vi "Main.vi"() -> ()   [LabVIEW 2019]
uses:
  Type defs/Elevator position.ctl
  Type defs/Car buttons.ctl
  Type defs/Main states.ctl
  Type defs/Elevator states.ctl
panel:
  in  "Select mode":bool
  in  "Floor array":cluster{"Up Button":bool, "Down Button":bool}[](array[cluster])
  in  "E4":T1
  in  "E3":T1
  in  "E2":T1
  in  "E1":T1
  in  "stop":bool
  # "20"
  # "19"
  # "18"
  # "17"
  # "16"
  # "15"
  # "14"
  # "13"
  # "12"
  # "11"
  # "10"
  # "9"
  # "8"
  # "7"
  # "6"
  # "5"
  # "4"
  # "3"
  # "2"
  # "1"
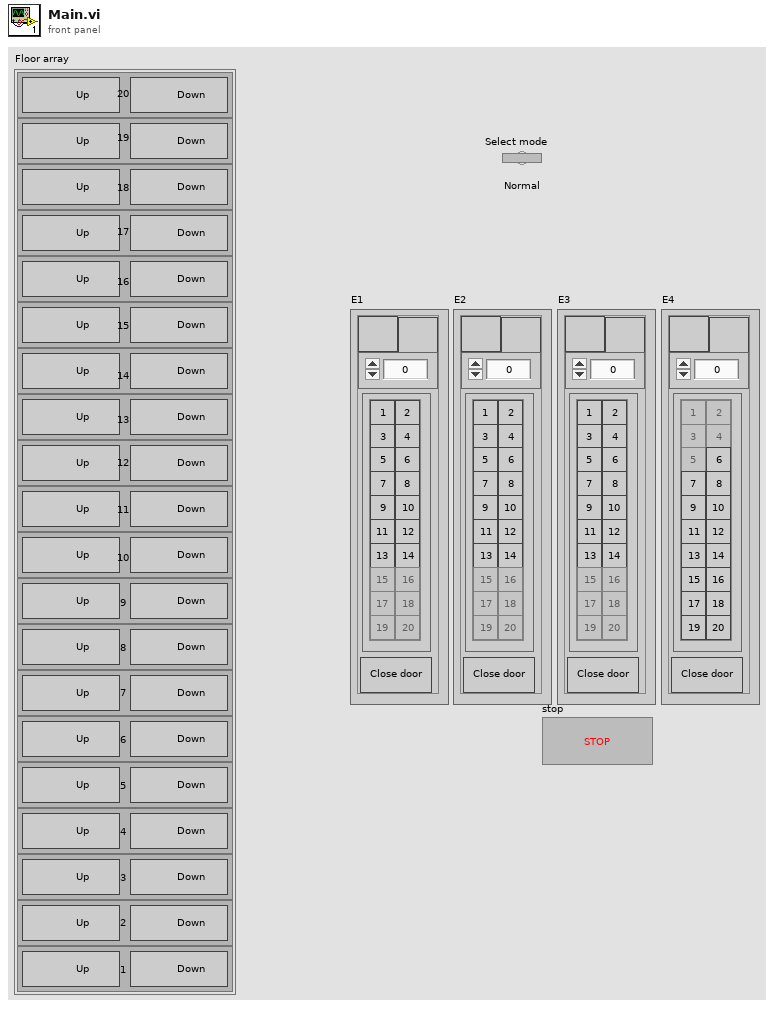
[diagram p1: front panel]
types:
  T1 = typedef "Elevator position.ctl" = cluster{"Up Button":bool, "Current floor":u16, "Down Button":bool, "Car":T2, "Close door":bool}
  T2 = typedef "Car buttons.ctl" = cluster{"Blank Button":bool, "Blank Button 2":bool, "Blank Button 3":bool, "Blank Button 4":bool, "Blank Button 5":bool, "Blank Button 6":bool, "Blank Button 7":bool, "Blank Button 8":bool, "Blank Button 9":bool, "Blank Button 10":bool, "Blank Button 11":bool, "Blank Button 12":bool, "Blank Button 13":bool, "Blank Button 14":bool, "Blank Button 15":bool, "Blank Button 16":bool, "Blank Button 17":bool, "Blank Button 18":bool, "Blank Button 19":bool, "Blank Button 20":bool}
  T3 = typedef "Main states.ctl" = enum16{"Init", "GUI", "Check next destination", "Move elevator", "Wait button press", "End"}
  T4 = typedef "Elevator states.ctl" = cluster{"Elevator":T1, "Destinations":i32[], "Idle floor":u16, "Max floor":u16, "Min floor":u16, "Next floor":u16, "Move started":timestamp, "Idle move":bool}
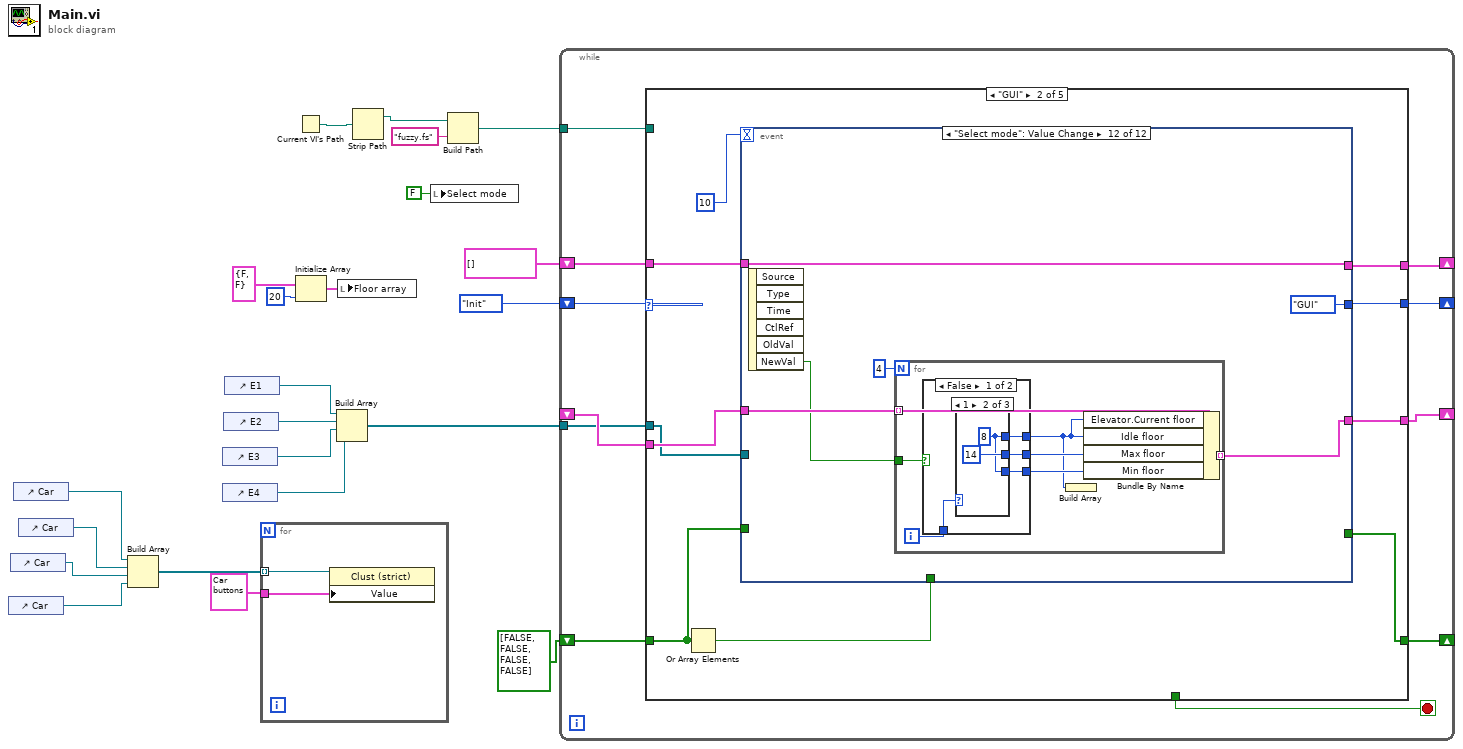
[diagram p0: block diagram]
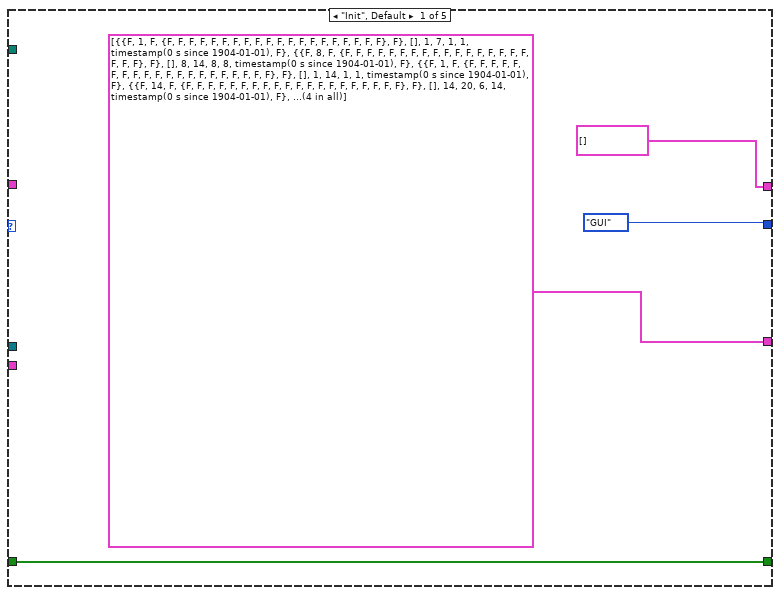
[diagram p2: hidden frame]
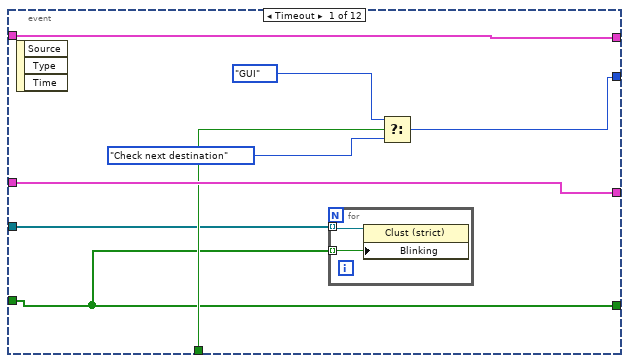
[diagram p3: hidden frame]
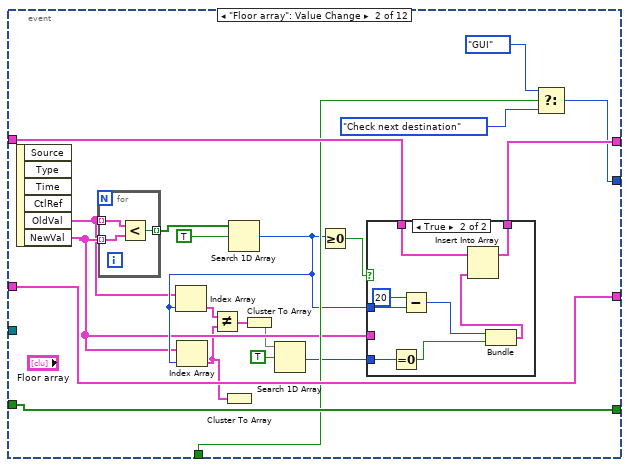
[diagram p4: hidden frame]
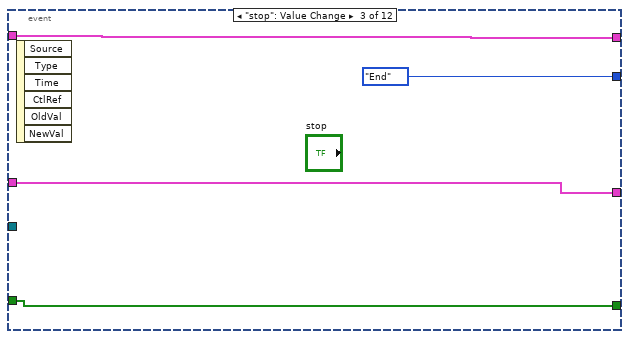
[diagram p6: hidden frame]
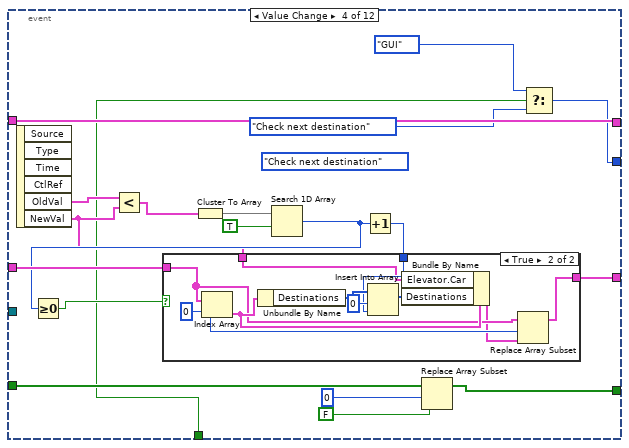
[diagram p7: hidden frame]
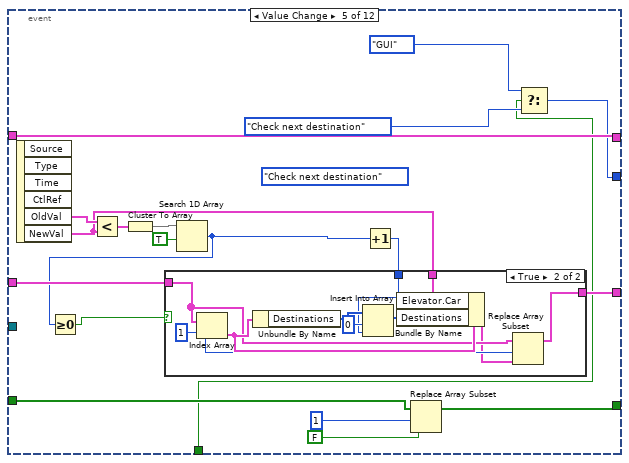
[diagram p9: hidden frame]
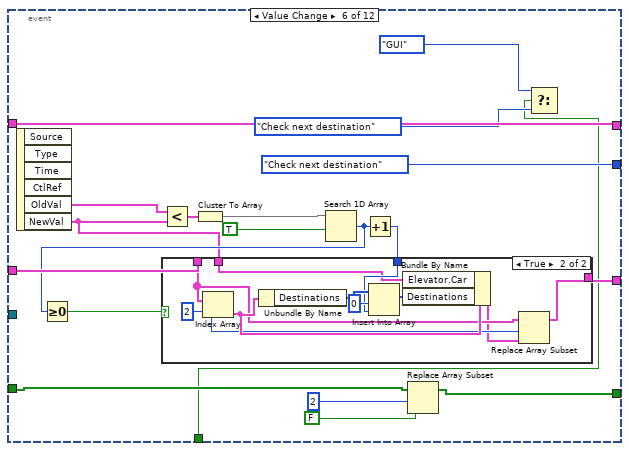
[diagram p11: hidden frame]
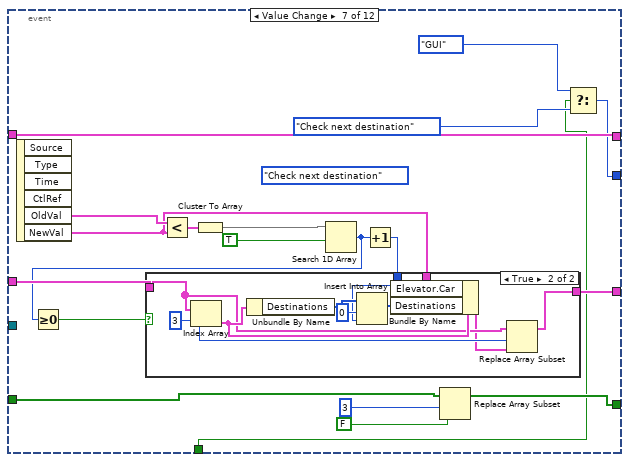
[diagram p13: hidden frame]
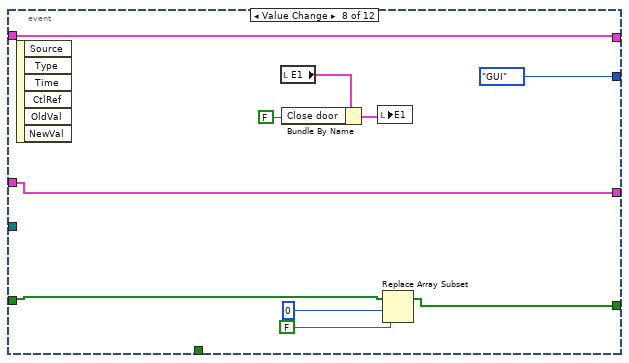
[diagram p15: hidden frame]
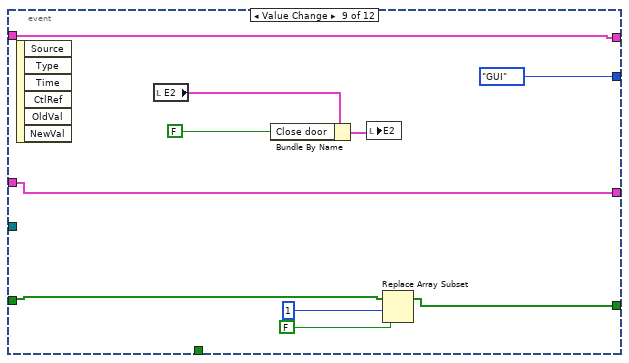
[diagram p16: hidden frame]
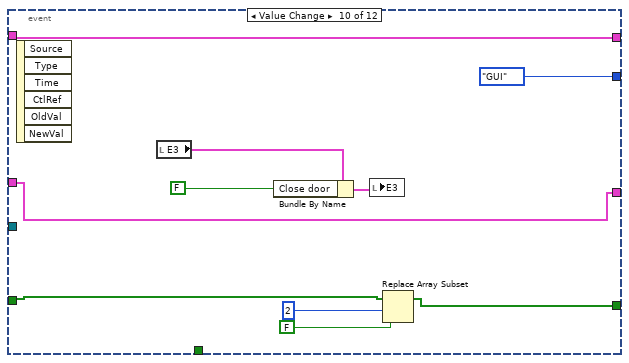
[diagram p17: hidden frame]
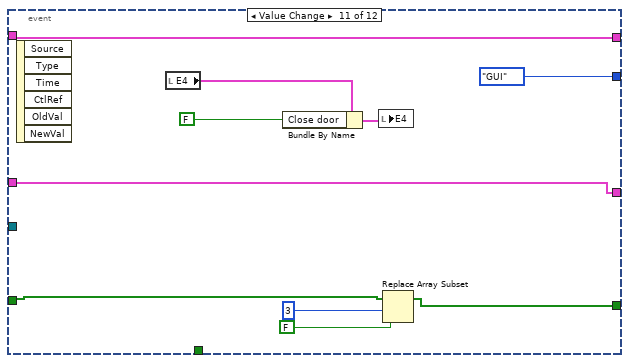
[diagram p18: hidden frame]
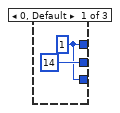
[diagram p19: hidden frame]
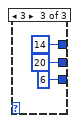
[diagram p20: hidden frame]
diagram:
  n1 = control-ref of="Car"() -> (w3:refnum<vi>)
  n2 = control-ref of="Car"() -> (w4:refnum<vi>)
  n3 = control-ref of="Car"() -> (w6:refnum<vi>)
  n4 = control-ref of="Car"() -> (w5:refnum<vi>)
  n5 = Build Array(w6, w5, w4, w3) -> (w2:refnum<vi>[])
  n6 = control-ref of="E3"() -> (w18:refnum<vi>)
  n7 = control-ref of="E4"() -> (w17:refnum<vi>)
  n8 = control-ref of="E2"() -> (w19:refnum<vi>)
  n9 = control-ref of="E1"() -> (w20:refnum<vi>)
  n10 = for {
    tunnel: T2 {"Blank Button"=FALSE, "Blank Button 2"=FALSE, "Blank Button 3"=FALSE, "Blank Button 4"=FALSE, "Blank Button 5"=FALSE, "Blank Button 6"=FALSE, "Blank Button 7"=FALSE, "Blank Button 8"=FALSE, "Blank Button 9"=FALSE, "Blank Button 10"=FALSE, "Blank Button 11"=FALSE, "Blank Button 12"=FALSE, "Blank Button 13"=FALSE, "Blank Button 14"=FALSE, "Blank Button 15"=FALSE, "Blank Button 16"=FALSE, "Blank Button 17"=FALSE, "Blank Button 18"=FALSE, "Blank Button 19"=FALSE, "Blank Button 20"=FALSE} ("Value") -> [w24]
    tunnel: w2 -> [w23] mode=indexing
    n11 = property class="Clust (strict)"(reference=w23, "Value"=w24) -> ()  [unwired: 1 in, 2 out]
  }
  n12 = Current VI's Path() -> (path=w12:path)
  n13 = Initialize Array(cluster{"Up Button":bool, "Down Button":bool} {"Up Button"=FALSE, "Down Button"=FALSE} ("Cluster"), 20 ("dimension size")) -> (w8:cluster{"Up Button":bool, "Down Button":bool}[])
  n14 = Build Array(w20, w19, w18, w17) -> (w16:refnum<vi>[])
  n15 = local write "Floor array"(w8) -> ()
  n16 = Strip Path(path=w12) -> (stripped path=w13:path)  [unwired: 1 out]
  n17 = local write "Select mode"(FALSE ("Select mode")) -> ()
  n18 = Build Path(base path=w13, name or relative path="fuzzy.fs") -> (appended path=w11:path)
  n19 = while {
    shift-right: [w34] -> _
    shift-left: cluster{"H call":dbl, "Up":bool}[] [] ("Array") -> [w33]
    shift-right: [w30] -> _
    shift-left: Main_states."Init" -> [w35]
    shift-right: [w29] -> _
    shift-left: _ -> [w32]
    tunnel: w16 -> [w28]
    shift-right: [w27] -> _
    shift-left: bool[] [FALSE, FALSE, FALSE, FALSE] ("Served car") -> [w26]
    tunnel: w11 -> [w25]
    stop <- w31 stop-if-true
    n20 = case shown="\"GUI\"" w35 {
      tunnel: [cluster{"H call":dbl, "Up":bool}[] [] ("Array") w48 w295 w327 w351] -> w34
      tunnel: w33 -> [_ w47 w296 w327 w351]
      tunnel: [Main_states."GUI" w46 Main_states."Move elevator" Main_states."GUI" Main_states."End"] -> w30
      tunnel: [T4[] [{"Elevator"={"Up Button"=FALSE, "Current floor"=1, "Down Button"=FALSE, "Car"={"Blank Button"=FALSE, "Blank Button 2"=FALSE, "Blank Button 3"=FALSE, "Blank Button 4"=FALSE, "Blank Button 5"=FALSE, "Blank Button 6"=FALSE, "Blank Button 7"=FALSE, "Blank Button 8"=FALSE, "Blank Button 9"=FALSE, "Blank Button 10"=FALSE, "Blank Button 11"=FALSE, "Blank Button 12"=FALSE, "Blank Button 13"=FALSE, "Blank Button 14"=FALSE, "Blank Button 15"=FALSE, "Blank Button 16"=FALSE, "Blank Button 17"=FALSE, "Blank Button 18"=FALSE, "Blank Button 19"=FALSE, "Blank Button 20"=FALSE}, "Close door"=FALSE}, "Destinations"=[], "Idle floor"=1, "Max floor"=7, "Min floor"=1, "Next floor"=1, "Move started"=timestamp(0 s since 1904-01-01), "Idle move"=FALSE}, {"Elevator"={"Up Button"=FALSE, "Current floor"=8, "Down Button"=FALSE, "Car"={"Blank Button"=FALSE, "Blank Button 2"=FALSE, "Blank Button 3"=FALSE, "Blank Button 4"=FALSE, "Blank Button 5"=FALSE, "Blank Button 6"=FALSE, "Blank Button 7"=FALSE, "Blank Button 8"=FALSE, "Blank Button 9"=FALSE, "Blank Button 10"=FALSE, "Blank Button 11"=FALSE, "Blank Button 12"=FALSE, "Blank Button 13"=FALSE, "Blank Button 14"=FALSE, "Blank Button 15"=FALSE, "Blank Button 16"=FALSE, "Blank Button 17"=FALSE, "Blank Button 18"=FALSE, "Blank Button 19"=FALSE, "Blank Button 20"=FALSE}, "Close door"=FALSE}, "Destinations"=[], "Idle floor"=8, "Max floor"=14, "Min floor"=8, "Next floor"=8, "Move started"=timestamp(0 s since 1904-01-01), "Idle move"=FALSE}, {"Elevator"={"Up Button"=FALSE, "Current floor"=1, "Down Button"=FALSE, "Car"={"Blank Button"=FALSE, "Blank Button 2"=FALSE, "Blank Button 3"=FALSE, "Blank Button 4"=FALSE, "Blank Button 5"=FALSE, "Blank Button 6"=FALSE, "Blank Button 7"=FALSE, "Blank Button 8"=FALSE, "Blank Button 9"=FALSE, "Blank Button 10"=FALSE, "Blank Button 11"=FALSE, "Blank Button 12"=FALSE, "Blank Button 13"=FALSE, "Blank Button 14"=FALSE, "Blank Button 15"=FALSE, "Blank Button 16"=FALSE, "Blank Button 17"=FALSE, "Blank Button 18"=FALSE, "Blank Button 19"=FALSE, "Blank Button 20"=FALSE}, "Close door"=FALSE}, "Destinations"=[], "Idle floor"=1, "Max floor"=14, "Min floor"=1, "Next floor"=1, "Move started"=timestamp(0 s since 1904-01-01), "Idle move"=FALSE}, {"Elevator"={"Up Button"=FALSE, "Current floor"=14, "Down Button"=FALSE, "Car"={"Blank Button"=FALSE, "Blank Button 2"=FALSE, "Blank Button 3"=FALSE, "Blank Button 4"=FALSE, "Blank Button 5"=FALSE, "Blank Button 6"=FALSE, "Blank Button 7"=FALSE, "Blank Button 8"=FALSE, "Blank Button 9"=FALSE, "Blank Button 10"=FALSE, "Blank Button 11"=FALSE, "Blank Button 12"=FALSE, "Blank Button 13"=FALSE, "Blank Button 14"=FALSE, "Blank Button 15"=FALSE, "Blank Button 16"=FALSE, "Blank Button 17"=FALSE, "Blank Button 18"=FALSE, "Blank Button 19"=FALSE, "Blank Button 20"=FALSE}, "Close door"=FALSE}, "Destinations"=[], "Idle floor"=14, "Max floor"=20, "Min floor"=6, "Next floor"=14, "Move started"=timestamp(0 s since 1904-01-01), "Idle move"=FALSE}] ("Elevator states array") w44 w294 w312 w350] -> w29
      tunnel: w32 -> [_ w45 w293 w325 w350]
      tunnel: [_ _ _ _ TRUE] -> w31
      tunnel: w28 -> [_ w40 _ _ _]
      tunnel: [w36 w41 w291 w309 w347] -> w27
      tunnel: w26 -> [w36 w42 w291 _ w347]
      tunnel: w25 -> [_ _ w289 _ _]
      frame "Init", Default {
      }
      frame "GUI" {
        n21 = Or Array Elements(Boolean array=w42) -> (logical OR=w43:bool)
        n22 = event shown="[11] \"Select mode\": Value Change" {
          selector: _ -> [_ _ _ _ _ _ _ _ _ _ _ _]
          dyn-events: _ -> [_ _ _ _ _ _ _ _ _ _ _ _]
          timeout: 10 -> [_ _ _ _ _ _ _ _ _ _ _ _]
          tunnel: [w57 w75 w95 w110 w140 w170 w200 w218 w228 w237 w251 w260] -> w48
          tunnel: w47 -> [w57 w76 w95 w110 w140 w170 w200 w218 w228 w237 w251 w260]
          tunnel: [w53 w70 Main_states."End" w96 w127 Main_states."Check next destination" w187 Main_states."GUI" Main_states."GUI" Main_states."GUI" Main_states."GUI" Main_states."GUI"] -> w46
          tunnel: w45 -> [w56 w79 w93 w108 w138 w167 w198 w217 w226 w238 w250 w259]
          tunnel: [w56 w79 w93 w107 w137 w166 w197 w217 w226 w238 w250 w257] -> w44
          tunnel: w43 -> [w55 w71 _ w97 w128 w157 w188 _ _ _ _ _]
          tunnel: w42 -> [w50 w74 w92 w103 w132 w161 w192 w223 w233 w243 w253 _]
          tunnel: [w50 w74 w92 w100 w131 w160 w191 w222 w232 w242 w252 _] -> w41
          tunnel: w40 -> [w51 _ _ _ _ _ _ _ _ _ _ _]
          event Timeout {
            n23 = event-data() -> ()  [unwired: 1 in, 3 out]
            n24 = for {
              tunnel: w51 -> [w59] mode=indexing
              tunnel: w50 -> [w58] mode=indexing
              n25 = property class="Clust (strict)"(reference=w59, "Blinking"=w58) -> ()  [unwired: 1 in, 2 out]
            }
            n26 = Select(t=Main_states."GUI", s=w55, f=Main_states."Check next destination") -> (s? t:f=w53:T3)
          }
          event "Floor array": Value Change {
            n27 = event-data() -> ("OldVal"=w63:cluster{"Up Button":bool, "Down Button":bool}[], "NewVal"=w68:cluster{"Up Button":bool, "Down Button":bool}[])  [unwired: 1 in, 4 out]
            n28 = for {
              tunnel: w63 -> [w91] mode=indexing
              tunnel: w68 -> [w90] mode=indexing
              tunnel: [w89] -> w78 mode=indexing
              n29 = Less?(x=w91, y=w90) -> (x < y?=w89:bool)
            }
            n30 = Search 1D Array(1D array=w78, element=TRUE) -> (index of element=w69:i32)  [unwired: 1 in]
            n31 = Index Array(array=w63, index=w69) -> (element=w67:cluster{"Up Button":bool, "Down Button":bool})
            n32 = Index Array(array=w68, index=w69) -> (element=w61:cluster{"Up Button":bool, "Down Button":bool})
            n33 = Not Equal?(x=w67, y=w61) -> (x != y?=w66:cluster{"Up Button":bool, "Down Button":bool})
            n34 = Cluster To Array(cluster=w61) -> ()  [unwired: 1 out]
            n35 = Cluster To Array(cluster=w66) -> (array=w62:bool[])
            n36 = Search 1D Array(1D array=w62, element=TRUE) -> (index of element=w60:i32)  [unwired: 1 in]
            n37 = Greater Or Equal To 0?(x=w69) -> (x >= 0?=w77:bool)
            n38 = case shown="True" w77 {
              tunnel: w69 -> [_ w88]
              tunnel: w76 -> [w80 w86]
              tunnel: [w80 w85] -> w75
              tunnel: w68 -> [_ _]
              tunnel: w60 -> [_ w82]
              frame False {
              }
              frame True {
                n39 = Equal To 0?(x=w82) -> (x = 0?=w81:bool)
                n40 = Subtract(x=20, y=w88) -> (x-y=w84:i32)
                n41 = Bundle(w84, w81) -> (w83:cluster{i32, bool})  [unwired: 1 in]
                n42 = Insert Into Array(array=w86, new element=w83) -> (w85:cluster{"H call":dbl, "Up":bool}[])  [unwired: 1 in]
              }
            }
            n43 = Select(t=Main_states."GUI", s=w71, f=Main_states."Check next destination") -> (s? t:f=w70:T3)
          }
          event "stop": Value Change {
            n44 = event-data() -> ()  [unwired: 1 in, 6 out]
          }
          event Value Change {
            (unwired) Main_states."Check next destination"
            n45 = event-data() -> ("OldVal"=w111:T2, "NewVal"=w104:T2)  [unwired: 1 in, 4 out]
            n46 = Less?(x=w111, y=w104) -> (x < y?=w114:T2)
            n47 = Cluster To Array(cluster=w114) -> (array=w113:bool[])
            n48 = Search 1D Array(1D array=w113, element=TRUE) -> (index of element=w106:i32)  [unwired: 1 in]
            n49 = Greater Or Equal To 0?(x=w106) -> (x >= 0?=w105:bool)
            n50 = Increment(x=w106) -> (x+1=w109:i32)
            n51 = case shown="True" w105 {
              tunnel: w109 -> [_ w122]
              tunnel: w108 -> [w115 w120]
              tunnel: [w115 w117] -> w107
              tunnel: w104 -> [_ w116]
              frame False {
              }
              frame True {
                w119 = 0 ("index")
                n52 = Index Array(array=w120, index=w119) -> (element=w125:T4)
                n53 = Unbundle By Name(w125) -> ("Destinations"=w124:i32[])
                n54 = Insert Into Array(array=w124, index=0, new element=w122) -> (w121:i32[])
                n55 = Bundle By Name(cluster=w125, "Elevator.Car"=w116, "Destinations"=w121) -> (w118:T4)
                n56 = Replace Array Subset(array=w120, new element=w118, index=w119) -> (w117:T4[])
              }
            }
            n57 = Replace Array Subset(array=w103, new element=FALSE ("new element/subarray"), index=0) -> (w100:bool[])
            n58 = Select(t=Main_states."GUI", s=w97, f=Main_states."Check next destination") -> (s? t:f=w96:T3)
          }
          event Value Change {
            (unwired) Main_states."Check next destination"
            n59 = event-data() -> ("OldVal"=w141:T2, "NewVal"=w126:T2)  [unwired: 1 in, 4 out]
            n60 = Less?(x=w141, y=w126) -> (x < y?=w144:T2)
            n61 = Cluster To Array(cluster=w144) -> (array=w143:bool[])
            n62 = Search 1D Array(1D array=w143, element=TRUE) -> (index of element=w136:i32)  [unwired: 1 in]
            n63 = Greater Or Equal To 0?(x=w136) -> (x >= 0?=w135:bool)
            n64 = Increment(x=w136) -> (x+1=w139:i32)
            n65 = case shown="True" w135 {
              tunnel: w139 -> [_ w152]
              tunnel: w138 -> [w145 w150]
              tunnel: [w145 w147] -> w137
              tunnel: w126 -> [_ w146]
              frame False {
              }
              frame True {
                w149 = 1 ("index")
                n66 = Index Array(array=w150, index=w149) -> (element=w155:T4)
                n67 = Unbundle By Name(w155) -> ("Destinations"=w154:i32[])
                n68 = Insert Into Array(array=w154, index=0, new element=w152) -> (w151:i32[])
                n69 = Bundle By Name(cluster=w155, "Elevator.Car"=w146, "Destinations"=w151) -> (w148:T4)
                n70 = Replace Array Subset(array=w150, new element=w148, index=w149) -> (w147:T4[])
              }
            }
            n71 = Replace Array Subset(array=w132, new element=FALSE ("new element/subarray"), index=1) -> (w131:bool[])
            n72 = Select(t=Main_states."GUI", s=w128, f=Main_states."Check next destination") -> (s? t:f=w127:T3)
          }
          event Value Change {
            n73 = event-data() -> ("OldVal"=w171:T2, "NewVal"=w156:T2)  [unwired: 1 in, 4 out]
            n74 = Less?(x=w171, y=w156) -> (x < y?=w174:T2)
            n75 = Cluster To Array(cluster=w174) -> (array=w173:bool[])
            n76 = Search 1D Array(1D array=w173, element=TRUE) -> (index of element=w164:i32)  [unwired: 1 in]
            n77 = Greater Or Equal To 0?(x=w164) -> (x >= 0?=w165:bool)
            n78 = Increment(x=w164) -> (x+1=w168:i32)
            n79 = case shown="True" w165 {
              tunnel: w168 -> [_ w182]
              tunnel: w167 -> [w175 w180]
              tunnel: [w175 w177] -> w166
              tunnel: w156 -> [_ w176]
              frame False {
              }
              frame True {
                w179 = 2 ("index")
                n80 = Index Array(array=w180, index=w179) -> (element=w185:T4)
                n81 = Unbundle By Name(w185) -> ("Destinations"=w184:i32[])
                n82 = Insert Into Array(array=w184, index=0, new element=w182) -> (w181:i32[])
                n83 = Bundle By Name(cluster=w185, "Elevator.Car"=w176, "Destinations"=w181) -> (w178:T4)
                n84 = Replace Array Subset(array=w180, new element=w178, index=w179) -> (w177:T4[])
              }
            }
            n85 = Replace Array Subset(array=w161, new element=FALSE ("new element/subarray"), index=2) -> (w160:bool[])
            n86 = Select(t=Main_states."GUI", s=w157, f=Main_states."Check next destination") -> ()  [unwired: 1 out]
          }
          event Value Change {
            (unwired) Main_states."Check next destination"
            n87 = event-data() -> ("OldVal"=w201:T2, "NewVal"=w186:T2)  [unwired: 1 in, 4 out]
            n88 = Less?(x=w201, y=w186) -> (x < y?=w204:T2)
            n89 = Cluster To Array(cluster=w204) -> (array=w203:bool[])
            n90 = Search 1D Array(1D array=w203, element=TRUE) -> (index of element=w195:i32)  [unwired: 1 in]
            n91 = Greater Or Equal To 0?(x=w195) -> (x >= 0?=w196:bool)
            n92 = Increment(x=w195) -> (x+1=w199:i32)
            n93 = case shown="True" w196 {
              tunnel: w199 -> [_ w212]
              tunnel: w198 -> [w205 w210]
              tunnel: [w205 w207] -> w197
              tunnel: w186 -> [_ w206]
              frame False {
              }
              frame True {
                w209 = 3 ("index")
                n94 = Index Array(array=w210, index=w209) -> (element=w215:T4)
                n95 = Unbundle By Name(w215) -> ("Destinations"=w214:i32[])
                n96 = Insert Into Array(array=w214, index=0, new element=w212) -> (w211:i32[])
                n97 = Bundle By Name(cluster=w215, "Elevator.Car"=w206, "Destinations"=w211) -> (w208:T4)
                n98 = Replace Array Subset(array=w210, new element=w208, index=w209) -> (w207:T4[])
              }
            }
            n99 = Replace Array Subset(array=w192, new element=FALSE ("new element/subarray"), index=3) -> (w191:bool[])
            n100 = Select(t=Main_states."GUI", s=w188, f=Main_states."Check next destination") -> (s? t:f=w187:T3)
          }
          event Value Change {
            n101 = event-data() -> ()  [unwired: 1 in, 6 out]
            n102 = local read "E1"() -> (w221:T1)
            n103 = Bundle By Name(cluster=w221, "Close door"=FALSE) -> (w219:T1)
            n104 = local write "E1"(w219) -> ()
            n105 = Replace Array Subset(array=w223, new element=FALSE ("new element/subarray"), index=0) -> (w222:bool[])
          }
          event Value Change {
            n106 = event-data() -> ()  [unwired: 1 in, 6 out]
            n107 = local read "E2"() -> (w231:T1)
            n108 = Bundle By Name(cluster=w231, "Close door"=FALSE) -> (w229:T1)
            n109 = local write "E2"(w229) -> ()
            n110 = Replace Array Subset(array=w233, new element=FALSE ("new element/subarray"), index=1) -> (w232:bool[])
          }
          event Value Change {
            n111 = event-data() -> ()  [unwired: 1 in, 6 out]
            n112 = local read "E3"() -> (w241:T1)
            n113 = Bundle By Name(cluster=w241, "Close door"=FALSE) -> (w239:T1)
            n114 = local write "E3"(w239) -> ()
            n115 = Replace Array Subset(array=w243, new element=FALSE ("new element/subarray"), index=2) -> (w242:bool[])
          }
          event Value Change {
            n116 = event-data() -> ()  [unwired: 1 in, 6 out]
            n117 = local read "E4"() -> (w248:T1)
            n118 = Bundle By Name(cluster=w248, "Close door"=FALSE) -> (w246:T1)
            n119 = local write "E4"(w246) -> ()
            n120 = Replace Array Subset(array=w253, new element=FALSE ("new element/subarray"), index=3) -> (w252:bool[])
          }
          event "Select mode": Value Change {
            n121 = event-data() -> ("NewVal"=w256:bool)  [unwired: 1 in, 5 out]
            n122 = for {
              N: 4 -> [_]
              tunnel: w259 -> [w268] mode=indexing
              tunnel: [w267] -> w257 mode=indexing
              tunnel: w256 -> [w266]
              i -> [w265]
              n123 = case shown="False" w266 {
                tunnel: w265 -> [w272 w283]
                tunnel: [w271 w282] -> w262
                tunnel: [w270 w281] -> w264
                tunnel: [w269 w280] -> w263
                frame False {
                  n124 = case shown="1" w272 {
                    tunnel: [w273 w275 u16 14 ("Idle floor")] -> w271
                    tunnel: [u16 14 ("Idle floor") u16 14 ("Idle floor") u16 20 ("Idle floor")] -> w270
                    tunnel: [w273 w275 u16 6 ("Idle floor")] -> w269
                    frame 0, Default {
                      w273 = u16 1 ("Idle floor")
                    }
                    frame 1 {
                      w275 = u16 8 ("Idle floor")
                    }
                    frame 3 {
                    }
                  }
                }
                frame True {
                  n125 = case shown="3" w283 {
                    tunnel: [w284 u16 14 ("Idle floor")] -> w282
                    tunnel: [u16 14 ("Idle floor") u16 20 ("Idle floor")] -> w281
                    tunnel: [w284 u16 6 ("Idle floor")] -> w280
                    frame 0, Default {
                      w284 = u16 1 ("Idle floor")
                    }
                    frame 3 {
                    }
                  }
                }
              }
              n126 = Build Array(w262) -> ()  [unwired: 1 out]
              n127 = Bundle By Name(cluster=w268, "Elevator.Current floor"=w262, "Idle floor"=w262, "Max floor"=w264, "Min floor"=w263) -> (w267:T4)
            }
          }
        }
      }
      frame "Check next destination" {
        n128 = case shown="True" "Select mode" {
          tunnel: w296 -> [w300 w308]
          tunnel: [w299 w307] -> w295
          tunnel: [w298 w306] -> w294
          tunnel: w293 -> [w297 w305]
          tunnel: w289 -> [_ w301]
          frame False {
            n129 = call "Normal mode logic.vi"("Elevator states array"=w297, "Floors to serve"=w300) -> ("Elevator states array out"=w298:T4[], "Floors to serve out"=w299:cluster{"H call":dbl, "Up":bool}[])  [unwired: 8 in]
          }
          frame True {
            n130 = call "Fuzzy logic.vi"("Floor height"=3.0, "Time per stop"=5, "Fuzzy system path"=w301, "Time per floor"=2, "Elevator states array"=w305, "Floors to serve"=w308) -> ("Elevator states array out"=w306:T4[], "Floors to serve out"=w307:cluster{"H call":dbl, "Up":bool}[])  [unwired: 4 in]
          }
        }
      }
      frame "Move elevator" {
        n131 = call "Next move 2.vi"("Elevator states in"=w325) -> ("Elevator states out"=w312:T4[], "Served floors"=w324:u16[], "Served car"=w309:bool[])  [unwired: 8 in]
        n132 = Build Array("E1", "E2", "E3", "E4") -> (w321:T1[])
        n133 = for {
          tunnel: w321 -> [w335] mode=indexing
          tunnel: w312 -> [w330] mode=indexing
          tunnel: [w328] -> w323 mode=indexing
          tunnel: w309 -> [w331] mode=indexing
          n134 = Unbundle By Name(w330) -> ("Elevator.Up Button"=w334:bool, "Elevator.Current floor"=w333:u16, "Elevator.Down Button"=w332:bool)
          n135 = Bundle By Name(cluster=w335, "Up Button"=w334, "Current floor"=w333, "Down Button"=w332) -> (w329:T1)
          n136 = case shown="True" w331 {
            tunnel: w330 -> [_ w340]
            tunnel: w329 -> [w336 w339]
            tunnel: [w336 w337] -> w328
            frame False {
            }
            frame True {
              n137 = Unbundle By Name(w340) -> ("Elevator.Car"=w338:T2)
              n138 = Bundle By Name(cluster=w339, "Car"=w338) -> (w337:T1)
            }
          }
        }
        n139 = local read "Floor array"() -> (w311:cluster{"Up Button":bool, "Down Button":bool}[])
        n140 = for {
          tunnel: w324 -> [w345] mode=indexing
          shift-right: [w342] -> w310
          shift-left: w311 -> [w346]
          n141 = Subtract(x=u16 20, y=w345) -> (x-y=w343:u16)
          n142 = Replace Array Subset(array=w346, new element=cluster{"Up Button":bool, "Down Button":bool} {"Up Button"=FALSE, "Down Button"=FALSE} ("new element/subarray"), index=w343) -> (w342:cluster{"Up Button":bool, "Down Button":bool}[])
        }
        n143 = Index Array(array=w323, index #1=0 ("index")) -> (element #1=w322:T1, element #2=w316:T1, element #3=w314:T1, element #4=w313:T1)  [unwired: 3 in]
        n144 = local write "Floor array"(w310) -> ()
        n145 = local write "E3"(w314) -> ()
        n146 = local write "E1"(w322) -> ()
        n147 = local write "E2"(w316) -> ()
        n148 = local write "E4"(w313) -> ()
      }
      frame "End" {
      }
    }
  }
